vi "What next.vi"   [LabVIEW 2010]
uses:
  SubVIs/LVPresent_Globals.vi
panel:
  # "Making your presentation"
  # "¥ once you have all your slides - move them around the way you want them\n¥ click on \"rebuild images\" - and that will update all the graphics\n¥ Select Define Bounce on a few slides and see what happens\n¥ Depress \"Select Order\" and then click on the slides in order\n\nTest with \"Preview\"\n\nPrint only works on a Mac - and it creates a pdf"
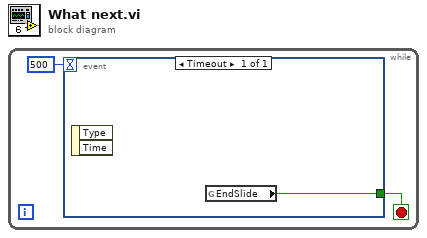
[diagram p0: block diagram]
diagram:
  n1 = while {
    stop <- w2 stop-if-true
    n2 = event shown="[0] Timeout" {
      selector: _ -> [_]
      dyn-events: _ -> [_]
      timeout: 500 -> [_]
      tunnel: [w3] -> w2
      event Timeout {
        n3 = event-data() -> ()  [unwired: 1 in, 2 out]
        n4 = global read "LVPresent_Globals.vi" "EndSlide"() -> (w3:bool)
      }
    }
  }
